vi "Read Power No Objects.vi"(8 "error in (no error)":errorcluster, 10 "VISA Resource Name":refnum<visa-resource-name>, 11 "Cluster In":T2={"Wavelength"=0.0, "AVG"=0, "Range"=0, "Backlight"=0, "Beeper"=0, "Zero"=0, "Local Lockout"=0, "ATTN"=0, "Run/Stop"=0, "Units"=0, "Averaging Points"=0, "Averaging"=FALSE, "Most Recent Power"=5.5, "Filter"=1} {"AVG" items=["Slow"=1, "Medium"=2, "Fast"=3]; "Range" items=["Auto", "Lowest", "2", "3", "4", "5", "6", "7", "Highest"]; "Backlight" items=["Off", "Low", "High"]; "Beeper" items=["Off", "On"]; "Zero" items=["Off", "On"]; "Local Lockout" items=["Off", "On"]; "ATTN" items=["Off", "On"]; "Run/Stop" items=["Stop", "Run"]; "Units" items=["W"=1, "dB"=2, "dBm"=3, "REL"=4]; "Filter" items=["Orange"=1, "Green"=2, "Yellow"=3]}) -> (0 "error out":errorcluster, 1 "Current Power w/ Units":string, 2 "Current Power":dbl[unit], 3 "Cluster Out":T2={"Wavelength"=0.0, "AVG"=0, "Range"=0, "Backlight"=0, "Beeper"=0, "Zero"=0, "Local Lockout"=0, "ATTN"=0, "Run/Stop"=0, "Units"=0, "Averaging Points"=0, "Averaging"=FALSE, "Most Recent Power"=5.5, "Filter"=1} {"AVG" items=["Slow"=1, "Medium"=2, "Fast"=3]; "Range" items=["Auto", "Lowest", "2", "3", "4", "5", "6", "7", "Highest"]; "Backlight" items=["Off", "Low", "High"]; "Beeper" items=["Off", "On"]; "Zero" items=["Off", "On"]; "Local Lockout" items=["Off", "On"]; "ATTN" items=["Off", "On"]; "Run/Stop" items=["Stop", "Run"]; "Units" items=["W"=1, "dB"=2, "dBm"=3, "REL"=4]; "Filter" items=["Orange"=1, "Green"=2, "Yellow"=3]})   [LabVIEW 2013]
doc: "Advanced Read for Power Meter.\n\nPerforms time-based Averaging based of member data. Checks for erroneous data points due to auto-ranging. Also has formatted power output."
uses:
  Public/Filters.ctl
  Newport 1830-C.lvlib
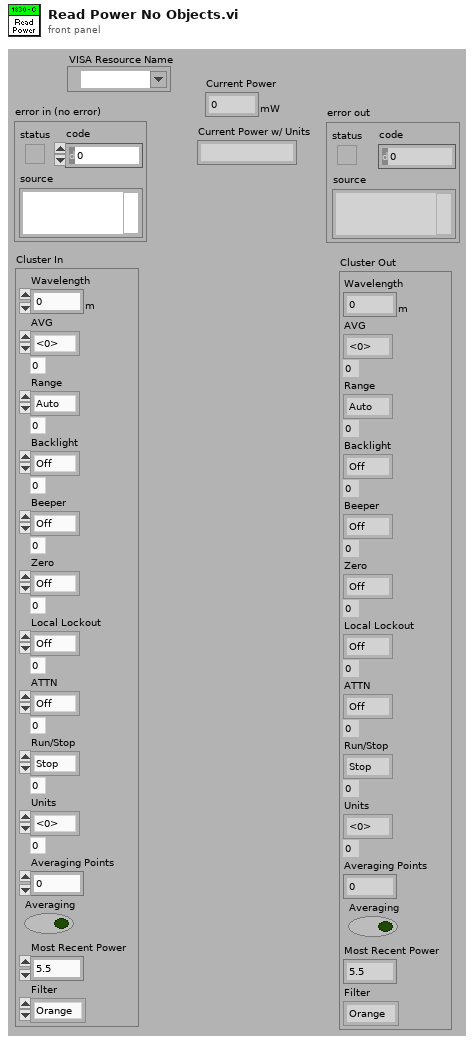
[diagram p1: front panel]
types:
  T1 = typedef "Newport 1830-C.lvlib/Filters.ctl" = u16
  T2 = cluster{"Wavelength":dbl[unit], "AVG":u16, "Range":u16, "Backlight":u16, "Beeper":u16, "Zero":u16, "Local Lockout":u16, "ATTN":u16, "Run/Stop":u16, "Units":u16, "Averaging Points":u32, "Averaging":bool, "Most Recent Power":dbl, "Filter":T1}
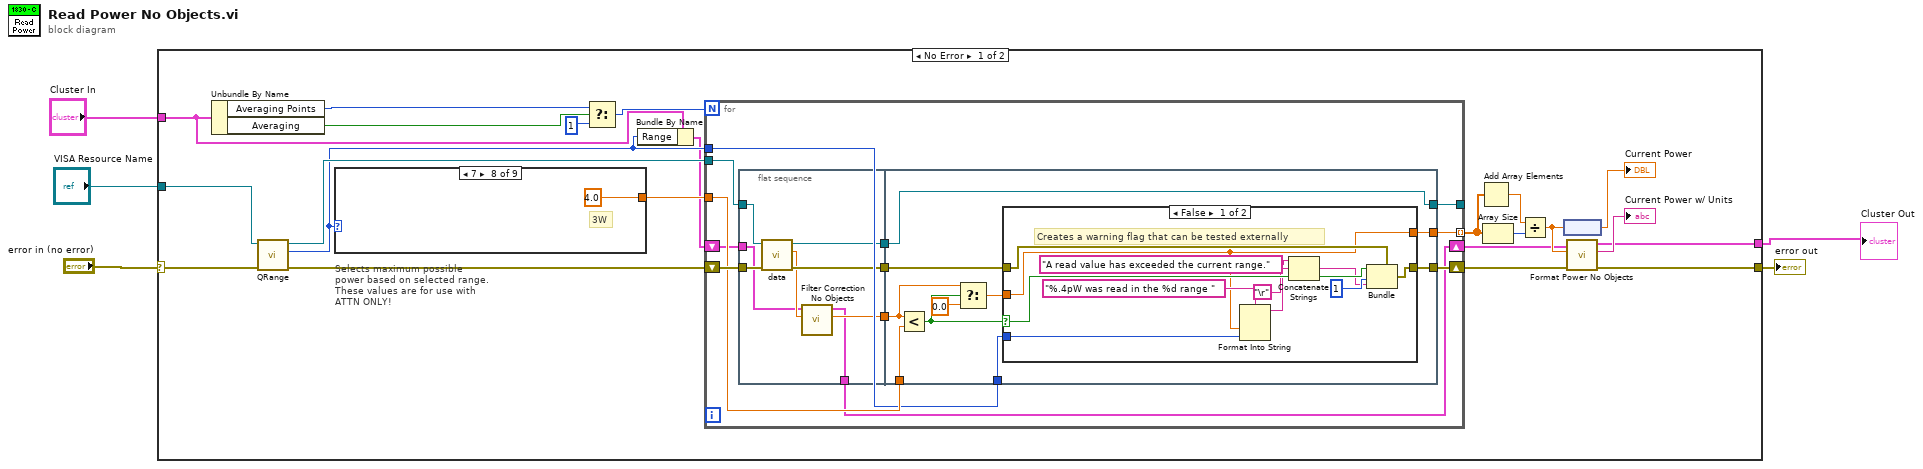
[diagram p0: block diagram]
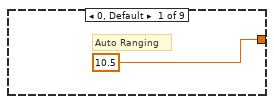
[diagram p2: hidden frame]
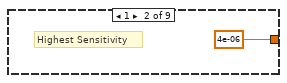
[diagram p3: hidden frame]
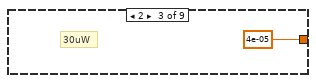
[diagram p4: hidden frame]
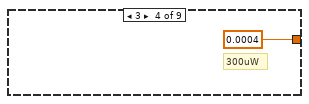
[diagram p5: hidden frame]
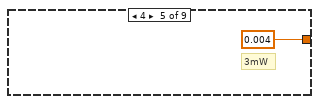
[diagram p6: hidden frame]
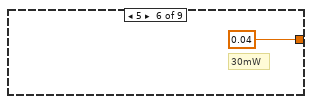
[diagram p7: hidden frame]
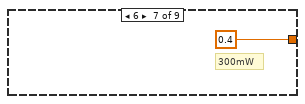
[diagram p8: hidden frame]
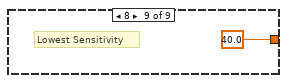
[diagram p9: hidden frame]
diagram:
  n1 = case shown="No Error" "error in (no error)" {
    selector: "error in (no error)" -> [w10 w81]
    tunnel: [w7 w81] -> w4
    tunnel: [w8 w80] -> w2
    tunnel: "VISA Resource Name" -> [w12 _]
    tunnel: "Cluster In" -> [w11 w80]
    frame No Error {
      n2 = Unbundle By Name(w11) -> ("Averaging Points"=w6:u32, "Averaging"=w22:bool)
      n3 = call "QRange.vi"("error in (no error)"=w10, "VISA resource name"=w12) -> ("error out"=w17:errorcluster, "Range"=w14:u32, "VISA resource name out"=w18:refnum<visa-resource-name>)  [unwired: 7 in]
      n4 = case "Selects maximum possible\npower based on selected range.\nThese values are for use with\nATTN ONLY!" shown="7" w14 {
        tunnel: [10.5 ("y") 4e-06 ("y") 4e-05 ("y") 0.0004 ("y") 0.004 ("y") 0.04 ("y") 0.4 ("y") 4.0 ("y") 40.0 ("y")] -> w16
        frame 0, Default {
          # "Auto Ranging"
        }
        frame 1 {
          # "Highest Sensitivity"
        }
        frame 2 {
          # "30uW"
        }
        frame 3 {
          # "300uW"
        }
        frame 4 {
          # "3mW"
        }
        frame 5 {
          # "30mW"
        }
        frame 6 {
          # "300mW"
        }
        frame 7 {
          # "3W"
        }
        frame 8 {
          # "Lowest Sensitivity"
        }
      }
      n5 = Select(t=w6, s=w22, f=u32 1 ("t")) -> (s? t:f=w23:u32)
      n6 = Bundle By Name(cluster=w11, "Range"=w14) -> (w13:T2)
      n7 = for {
        N: w23 -> [_]
        tunnel: w18 -> [w48]
        tunnel: [w46] -> _
        tunnel: w16 -> [w41]
        tunnel: w14 -> [w40]
        tunnel: [w39] -> w15 mode=indexing
        shift-right: [w45] -> w21
        shift-left: w17 -> [w47]
        shift-right: [w37] -> w9
        shift-left: w13 -> [w38]
        n8 = flat-sequence {
          tunnel: w48 -> [w56]
          tunnel: w47 -> [w55]
          tunnel: [w54] -> w44
          tunnel: [w53] -> w43
          tunnel: [w51] -> w42
          tunnel: w38 -> [w49]
          tunnel: [w50] -> w37
          tunnel: [w63] -> w45
          tunnel: [w66] -> w46
          tunnel: w44 -> [w66]
          tunnel: w43 -> [w64]
          tunnel: w42 -> [w61]
          tunnel: w41 -> [w62]
          tunnel: w40 -> [w59]
          tunnel: [w58] -> w39
          frame #0 {
            n9 = call "data.vi"("error in (no error)"=w55, "VISA resource name"=w56) -> ("error out"=w53:errorcluster, "Power"=w52:dbl, "VISA resource name out"=w54:refnum<visa-resource-name>)  [unwired: 7 in]
            n10 = call "Filter Correction No Objects.vi"("Read Power"=w52, "Cluster In"=w49) -> ("Corrected Power"=w51:dbl, "Cluster Out"=w50:T2)  [unwired: 8 in]
          }
          frame #1 {
            n11 = Less?(x=w61, y=w62) -> (x < y?=w57:bool)
            n12 = Select(t=w61, s=w57, f=0.0) -> (s? t:f=w60:dbl)
            n13 = case shown="False" w57 {
              selector: w57 -> [w76 _]
              tunnel: w64 -> [w77 w79]
              tunnel: [w74 w79] -> w63
              tunnel: w60 -> [w69 w78]
              tunnel: w59 -> [w70 _]
              tunnel: [w69 w78] -> w58
              frame False {
                # "Creates a warning flag that can be tested externally"
                n14 = Format Into String(format string="%.4pW was read in the %d range ", w69, w70) -> (resulting string=w68:string)  [unwired: 2 in, 1 out]
                n15 = Concatenate Strings("A read value has exceeded the current range." ("source"), "\r", w68) -> (w71:string)
                n16 = Bundle(cluster=w77, "status"=w76, "code"=1, "source"=w71) -> (w74:errorcluster)
              }
              frame True {
              }
            }
          }
        }
      }
      n17 = Add Array Elements(numeric array=w15) -> (sum=w25:dbl)
      n18 = Array Size(array=w15) -> (size(s)=w26:i32)
      n19 = Divide(x=w25, y=w26) -> (x/y=w20:dbl)
      n20 = node(w20) -> (→"Current Power":dbl[unit])
      n21 = call "Format Power No Objects.vi"("error in"=w21, "Power"=w20, "Cluster In"=w9) -> ("error out"=w7:errorcluster, "Formatted Power"=→"Current Power w/ Units":string, "Cluster Out"=w8:T2)  [unwired: 6 in]
    }
    frame Error {
    }
  }
  "error out" <- w4
  "Cluster Out" <- w2
